vi "close.vi"(8 "error in":errorcluster, 11 "TDMS datalogger runtime in":refnum<class "TDMS datalogger runtime.lvclass">) -> (0 "error out":errorcluster)   [LabVIEW 2013, in "TDMS datalogger runtime.lvclass"]
doc: "Provides an interface for terminating a module instance. While this interface performs no operations, a child should close and deallocate any open references or memory."
uses:
  TDMS datalogger runtime.lvclass
  control enum.ctl
  TDMS datalogger runtime.lvclass/TDMS datalogger runtime.ctl
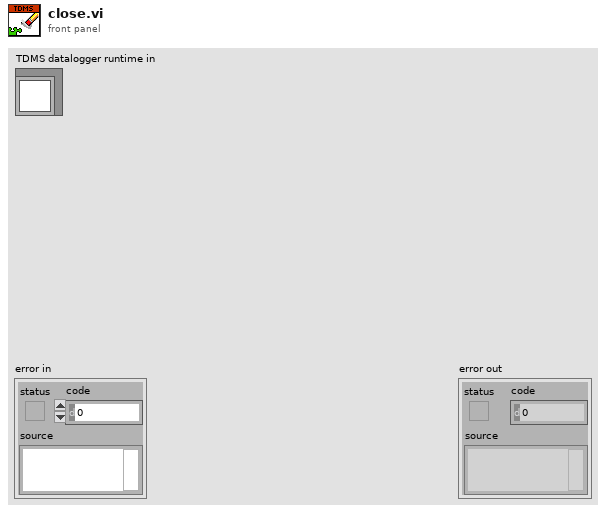
[diagram p1: front panel]
types:
  T1 = typedef "TDMS datalogger runtime.lvclass/control enum.ctl" = enum16{"exit"}
  T2 = typedef "TDMS datalogger runtime.lvclass/sample queue.ctl" = cluster{"data to processor":refnum<queue>, "time to processor":refnum<queue>}
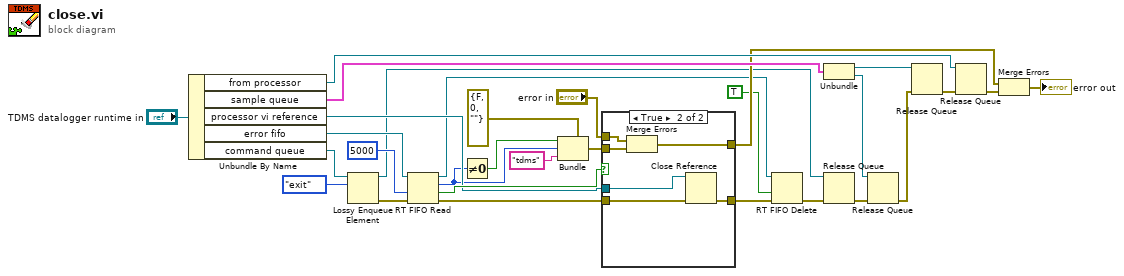
[diagram p0: block diagram]
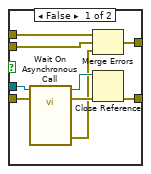
[diagram p2: hidden frame]
diagram:
  n1 = Unbundle By Name("TDMS datalogger runtime in") -> ("from processor"=w23:refnum<queue>, "sample queue"=w25:T2, "processor vi reference"=w26:refnum<vi>, "error fifo"=w30:refnum<k33>, "command queue"=w18:refnum<queue>)
  n2 = Lossy Enqueue Element(queue=w18, element=control_enum."exit") -> (queue out=w16:refnum<queue>, error out=w11:errorcluster)  [unwired: 1 in, 2 out]
  n3 = RT FIFO Read(0:w30, 2:5000 ("timeout in ms (-1)"), 3:w11) -> (8:w7:refnum<k33>, 9:w3:i32, 10:w28:bool, 11:w27:errorcluster)  [unwired: 1 in, 1 out]
  n4 = Not Equal To 0?(x=w3) -> (x != 0?=w5:bool)
  n5 = Bundle(cluster=errorcluster {"status"=FALSE, "code"=0, "source"=""} ("error out"), "status"=w5, "code"=w3, "source"="tdms") -> (w1:errorcluster)
  n6 = case shown="True" w28 {
    tunnel: w27 -> [w33 w43]
    tunnel: w26 -> [w34 w44]
    tunnel: w1 -> [w39 w45]
    tunnel: [w38 w41] -> w22
    tunnel: [w37 w42] -> w8
    tunnel: "error in" -> [w31 w40]
    frame False {
      n7 = call-by-ref "Wait On Asynchronous Call"(reference=w34, error in=w33) -> (reference out=w36:refnum<vi>, error out=w35:errorcluster, 19:"error out"=w32:errorcluster)  [unwired: 19 in]
      n8 = Merge Errors(w31, w39, w32) -> (w38:errorcluster)
      n9 = Close Reference(reference=w36, error in (no error)=w35) -> (error out=w37:errorcluster)
    }
    frame True {
      n10 = Merge Errors(w40, w45) -> (w41:errorcluster)
      n11 = Close Reference(reference=w44, error in (no error)=w43) -> (error out=w42:errorcluster)
    }
  }
  n12 = RT FIFO Delete(0:w7, 2:TRUE ("force destroy? (F)"), 3:w8) -> (11:w9:errorcluster)
  n13 = Unbundle(w25) -> ("data to processor"=w13:refnum<queue>, "time to processor"=w12:refnum<queue>)
  n14 = Release Queue(queue=w16, error in (no error)=w9) -> (error out=w15:errorcluster)  [unwired: 1 in, 2 out]
  n15 = Release Queue(queue=w12, error in (no error)=w15) -> (error out=w14:errorcluster)  [unwired: 1 in, 2 out]
  n16 = Release Queue(queue=w13, error in (no error)=w14) -> (error out=w24:errorcluster)  [unwired: 1 in, 2 out]
  n17 = Release Queue(queue=w23, error in (no error)=w24) -> (error out=w21:errorcluster)  [unwired: 1 in, 2 out]
  n18 = Merge Errors(w22, w21) -> (→"error out":errorcluster)
